vi "Read Device Information.vi"(8 "error in (no error)":errorcluster, 11 "TwinCAT ADS in":refnum<class "TwinCAT ADS.lvclass">) -> (0 "error out":errorcluster, 1 "Device Information":T1, 3 "TwinCAT ADS out":refnum<class "TwinCAT ADS.lvclass">)   [LabVIEW 2018, in "TwinCAT ADS.lvclass"]
uses:
  TwinCAT ADS.lvclass
  Controls/Device Information.ctl
  TwinCAT ADS.lvclass/TwinCAT ADS.ctl
  TwinCAT.Ads
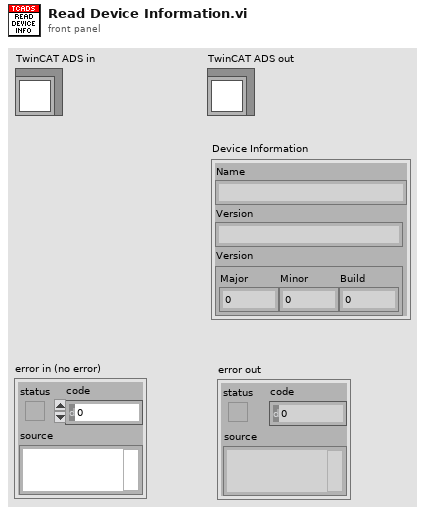
[diagram p1: front panel]
types:
  T1 = typedef "TwinCAT ADS.lvclass/Device Information.ctl" = cluster{"Name":string, "Version":string, "Version":cluster{"Major":i32, "Minor":i32, "Build":i32}}
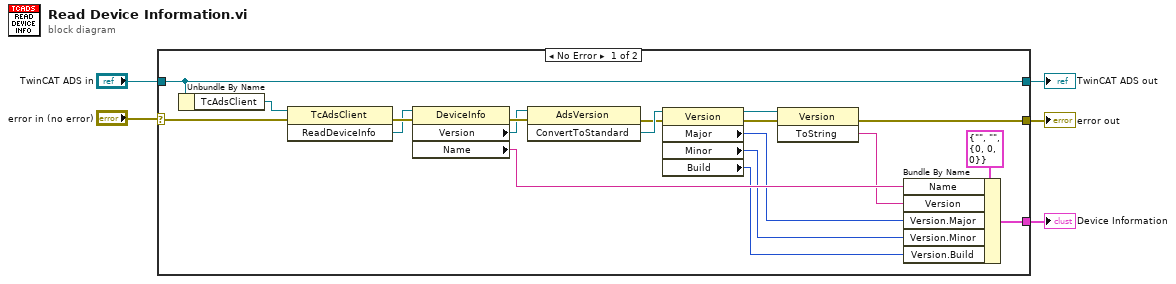
[diagram p0: block diagram]
diagram:
  n1 = case shown="No Error" "error in (no error)" {
    selector: "error in (no error)" -> [w20 w26]
    tunnel: [w7 w26] -> w4
    tunnel: [w24 w25] -> w2
    tunnel: "TwinCAT ADS in" -> [w24 w25]
    tunnel: [w6 _] -> w1
    frame No Error {
      n2 = Unbundle By Name(w24) -> ("TcAdsClient"=w21:refnum<k24>)
      n3 = invoke class="TcAdsClient" method="ReadDeviceInfo"(reference=w21, error in=w20) -> (error out=w23:errorcluster, "ReadDeviceInfo"=w22:refnum<k24>)  [unwired: 1 in, 1 out]
      n4 = property class="DeviceInfo"(reference=w22, error in=w23) -> (error out=w19:errorcluster, "Version"=w18:refnum<k24>, "Name"=w12:string)  [unwired: 1 out]
      n5 = invoke class="AdsVersion" method="ConvertToStandard"(reference=w18, error in=w19) -> (error out=w16:errorcluster, "ConvertToStandard"=w17:refnum<k24>)  [unwired: 1 in, 1 out]
      n6 = property class="Version"(reference=w17, error in=w16) -> (reference out=w14:refnum<k24>, error out=w15:errorcluster, "Major"=w10:i32, "Minor"=w9:i32, "Build"=w8:i32)
      n7 = invoke class="Version" method="ToString"(reference=w14, error in=w15) -> (error out=w7:errorcluster, "ToString"=w11:string)  [unwired: 1 in, 1 out]
      n8 = Bundle By Name(cluster=T1 {"Name"="", "Version"="", "Version"={"Major"=0, "Minor"=0, "Build"=0}} ("Device Infomation"), "Name"=w12, "Version"=w11, "Version.Major"=w10, "Version.Minor"=w9, "Version.Build"=w8) -> (w6:T1)
    }
    frame Error {
    }
  }
  "error out" <- w4
  "TwinCAT ADS out" <- w2
  "Device Information" <- w1
